vi "Test DQMH Power Requests API.vi"() -> ()   [LabVIEW 2024]
doc: "DQMH Power Requests API Tester.\n\n<b>Note:</b> This VI was modified by the <b>Validate DQMH Module</b> tool to upgrade it to the DQMH 5.0 approach to only call the Stop Module.vi at the end of the tester if the module wasn't originally running when the tester started.\n\n<b>Note:</b> This VI was modified by the <b>Validate DQMH Module</b> tool to add the 'Show Main VI Diagram on Init' functionality included in DQMH 6.1.\n\n<b>Note:</b> This VI was modified by the <b>Validate DQMH Module</b> tool to upgrade its Error Reported event frame to use an improved mechanism for displaying error information.\n\n<b>Note:</b> This VI was modified by the <b>Validate DQMH Module</b> tool to remove code to stop the main loop on error, and instead display the most recent error on the tester front panel."
uses:
  <vilib>/Utility/error.llb/DialogType.ctl
  DQMH Power Requests.lvlib
panel:
  out "last error":errorcluster
  in  "Show Main VI Diagram on Init (F)":bool
  in  "Display Required":bool
  in  "System Required":bool
  in  "Create Request":bool
  in  "Show Block Diagram":bool
  in  "Stop Module":bool
  in  "Start Module":bool
  in  "Hide Module Panel":bool
  in  "Show Module Panel":bool
  out "Status":string
  out "Module Running?":bool
  # "This VI tests the API for the Module."
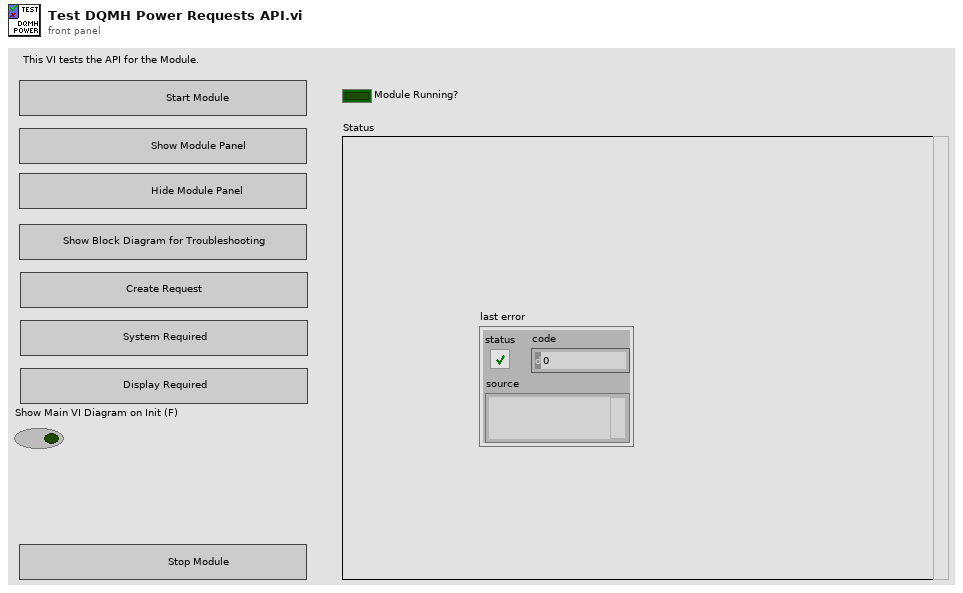
[diagram p1: front panel]
types:
  T1 = typedef "DQMH Power Requests.lvlib/Broadcast Events--cluster.ctl" = cluster{"Module Did Init":refnum<user-event>, "Status Updated":refnum<user-event>, "Error Reported":refnum<user-event>, "Module Did Stop":refnum<user-event>, "Update Module Execution Status":refnum<user-event>}
  T2 = typedef "DialogType.ctl" = u16
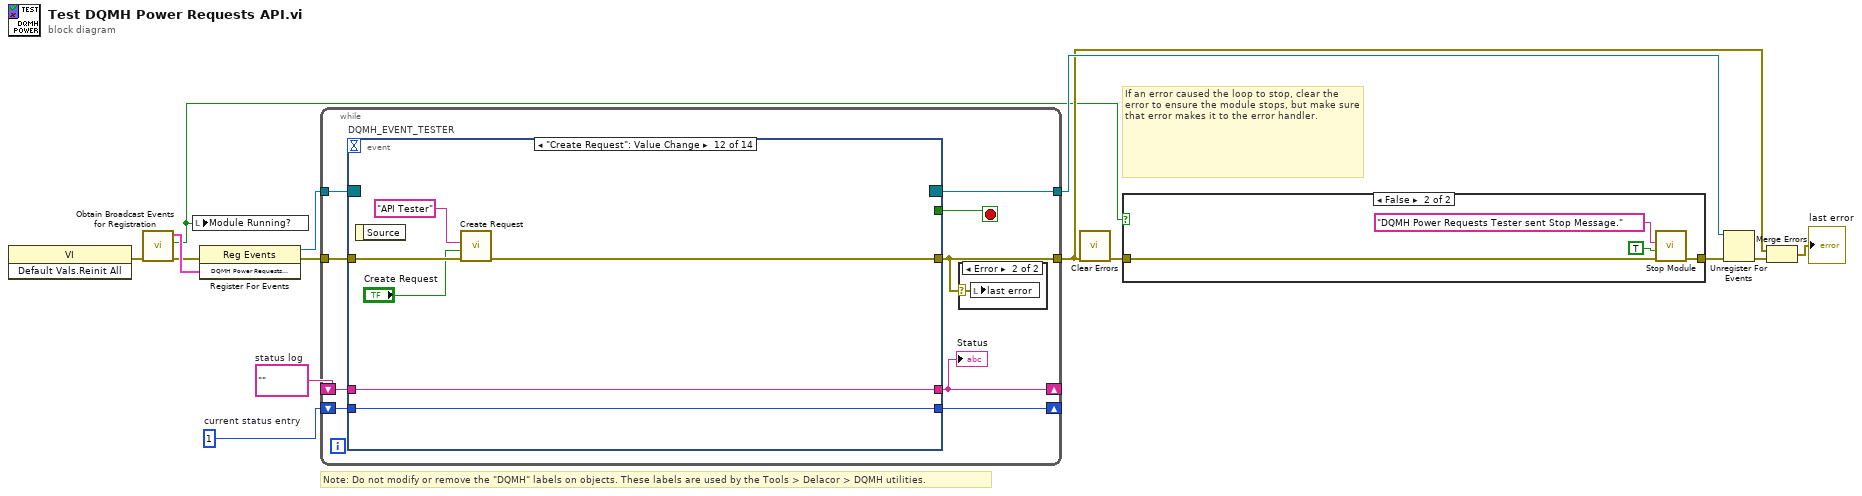
[diagram p0: block diagram]
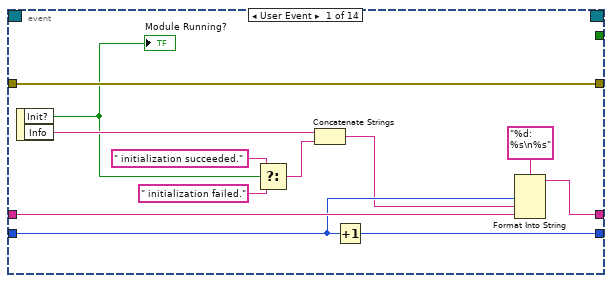
[diagram p4: hidden frame]
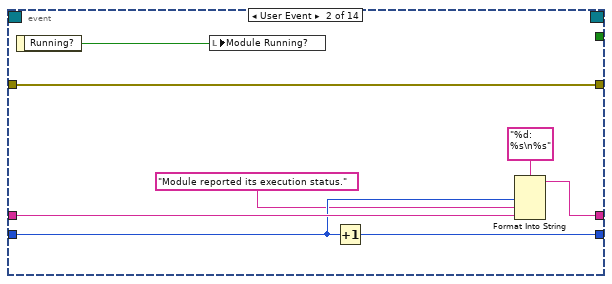
[diagram p5: hidden frame]
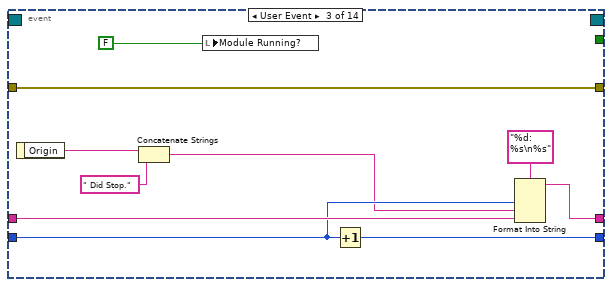
[diagram p6: hidden frame]
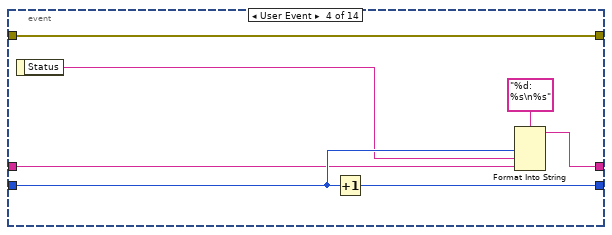
[diagram p7: hidden frame]
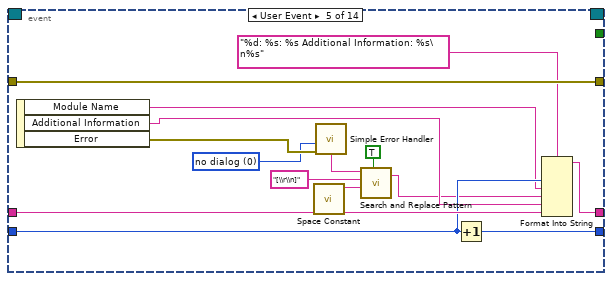
[diagram p8: hidden frame]
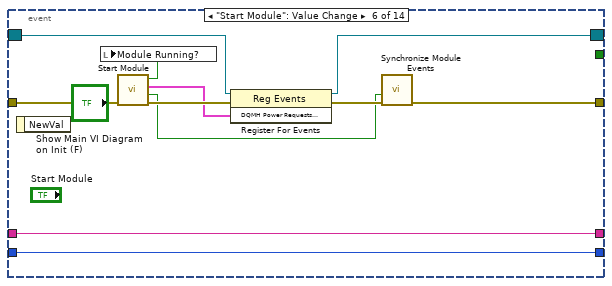
[diagram p9: hidden frame]
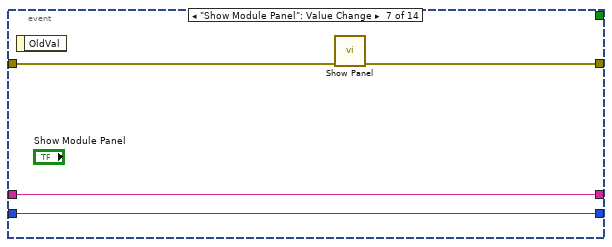
[diagram p10: hidden frame]
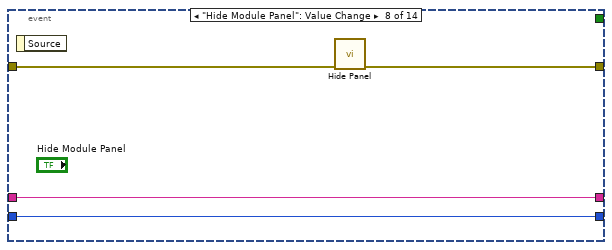
[diagram p11: hidden frame]
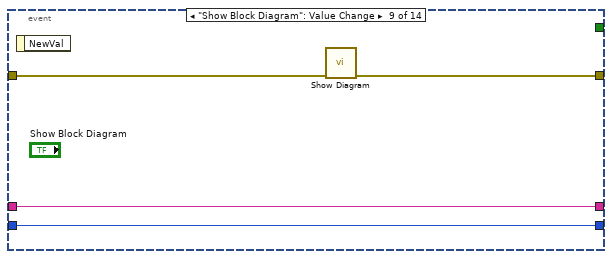
[diagram p12: hidden frame]
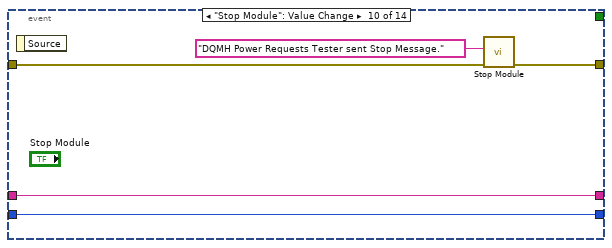
[diagram p13: hidden frame]
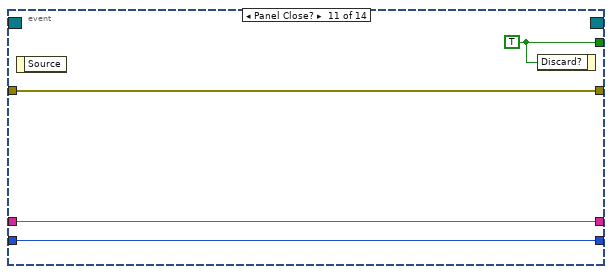
[diagram p14: hidden frame]
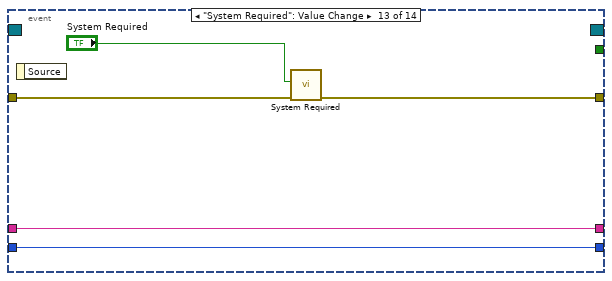
[diagram p15: hidden frame]
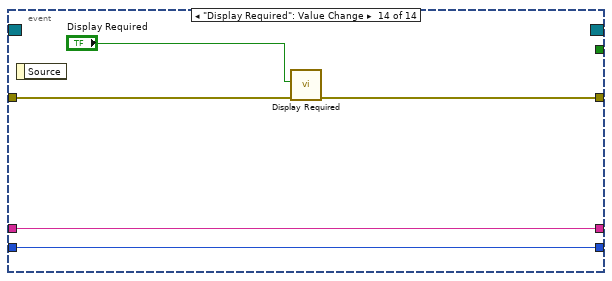
[diagram p16: hidden frame]
diagram:
  w11 = 1  # current status entry
  w12 = ""  # status log
  # "If an error caused the loop to stop, clear the error to ensure the module stops, but make sure that error makes it to the error handler."
  # "Note: Do not modify or remove the \"DQMH\" labels on objects. These labels are used by the Tools > Delacor > DQMH utilities."
  n1 = invoke class="VI" method="Default Vals.Reinit All"() -> (error out=w3:errorcluster)  [unwired: 3 in, 2 out]
  n2 = call "Obtain Broadcast Events for Registration.vi"("error in (no error)"=w3) -> ("error out"=w2:errorcluster, "Already running?"=w4:bool, "DQMH Power Requests Broadcast Events"=w9:T1)  [unwired: 8 in]
  n3 = local write "Module Running?"(w4) -> ()
  n4 = register-events(error in=w2, w9) -> (reference out=w8:refnum<event-registration>, error out=w10:errorcluster)  [unwired: 1 in]
  n5 = while {
    tunnel: w8 -> [w23]
    tunnel: [w16] -> w5
    shift-right: [w19] -> _
    shift-left: w12 -> [w21]
    shift-right: [w20] -> _
    shift-left: w11 -> [w22]
    tunnel: w10 -> [w18]
    tunnel: [w17] -> w7
    stop <- w15 stop-if-true
    n6 = event "DQMH_EVENT_TESTER" shown="[11] \"Create Request\": Value Change" {
      selector: w23 -> [_ _ _ _ _ w82 _ _ _ _ _ _ _ _]
      dyn-events: [_ _ _ _ _ w81 _ _ _ _ _ _ _ _] -> w17
      timeout: _ -> [_ _ _ _ _ _ _ _ _ _ _ _ _ _]
      tunnel: [_ _ _ _ _ _ _ _ _ _ w109 _ _ _] -> w15
      tunnel: [w36 w38 w45 w55 w76 w80 w92 w96 w97 w103 w106 w110 w117 w122] -> w16
      tunnel: w22 -> [w33 w42 w52 w58 w73 w85 w90 w94 w98 w104 w107 w113 w118 w123]
      tunnel: w21 -> [w34 w43 w53 w57 w75 w86 w91 w95 w99 w105 w108 w114 w119 w124]
      tunnel: [w31 w40 w50 w59 w74 w86 w91 w95 w99 w105 w108 w114 w119 w124] -> w19
      tunnel: [w32 w41 w51 w61 w72 w85 w90 w94 w98 w104 w107 w113 w118 w123] -> w20
      tunnel: w18 -> [w36 w38 w45 w55 w76 w79 w89 w93 w100 w101 w106 w115 w120 w125]
      event User Event {
        n7 = event-data() -> ("Init?"=w28:bool, "Info"=w30:string)  [unwired: 1 in]
        "Module Running?" <- w28
        n8 = Select(t=" initialization succeeded.", s=w28, f=" initialization failed.") -> (s? t:f=w25:string)
        n9 = Concatenate Strings(w30, w25) -> (w29:string)
        n10 = Increment(x=w33) -> (x+1=w32:i32)
        n11 = Format Into String(format string="%d: %s\n%s", w33, w29, w34) -> (resulting string=w31:string)  [unwired: 2 in, 1 out]
      }
      event User Event {
        n12 = event-data() -> ("Running?"=w37:bool)  [unwired: 1 in]
        n13 = local write "Module Running?"(w37) -> ()
        n14 = Increment(x=w42) -> (x+1=w41:i32)
        n15 = Format Into String(format string="%d: %s\n%s", w42, "Module reported its execution status.", w43) -> (resulting string=w40:string)  [unwired: 2 in, 1 out]
      }
      event User Event {
        n16 = event-data() -> ("Origin"=w49:string)  [unwired: 1 in]
        n17 = Concatenate Strings(w49, " Did Stop.") -> (w48:string)
        n18 = local write "Module Running?"(FALSE ("Module Did Init?")) -> ()
        n19 = Increment(x=w52) -> (x+1=w51:i32)
        n20 = Format Into String(format string="%d: %s\n%s", w52, w48, w53) -> (resulting string=w50:string)  [unwired: 2 in, 1 out]
      }
      event User Event {
        n21 = event-data() -> ("Status"=w56:string)  [unwired: 1 in]
        n22 = Increment(x=w58) -> (x+1=w61:i32)
        n23 = Format Into String(format string="%d: %s\n%s", w58, w56, w57) -> (resulting string=w59:string)  [unwired: 2 in, 1 out]
      }
      event User Event {
        w68 = T2 0 items=["no dialog", "OK message", "continue or stop message", "OK message + warnings", "continue/stop + warnings"] ("type of dialog (OK msg:1)")
        n24 = event-data() -> ("Module Name"=w69:string, "Additional Information"=w70:string, "Error"=w71:errorcluster)  [unwired: 1 in]
        n25 = call <vilib>:"Space Constant.vi"() -> ("String"=w64:string)
        n26 = call <vilib>:"Simple Error Handler.vi"("type of dialog (OK msg:1)"=w68, "error in (no error)"=w71) -> ("message"=w67:string)  [unwired: 3 in, 4 out]
        n27 = call <vilib>:"Search and Replace Pattern.vi"("string"=w67, "regular expression (\"\")"="[\\r\\n]" ("regular expression (\"\")"), "replace string (\"\")"=w64, "replace all? (F)"=TRUE ("replace all CR/LF with spaces")) -> ("result string"=w66:string)  [unwired: 1 in, 1 out]
        n28 = Increment(x=w73) -> (x+1=w72:i32)
        n29 = Format Into String(format string="%d: %s: %s Additional Information: %s\n%s", w73, w69, w66, w70, w75) -> (resulting string=w74:string)  [unwired: 2 in, 1 out]
      }
      event "Start Module": Value Change {
        n30 = event-data() -> ()  [unwired: 1 in, 1 out]
        n31 = call "Start Module.vi"("Show Main VI Diagram on Init (F)"="Show Main VI Diagram on Init (F)", "error in (no error)"=w79) -> ("error out"=w87:errorcluster, "Wait for Event Sync?"=w84:bool, "DQMH Power Requests Broadcast Events"=w83:T1, "Module Was Already Running?"=w78:bool)  [unwired: 6 in]
        n32 = local write "Module Running?"(w78) -> ()
        n33 = register-events(reference=w82, error in=w87, w83) -> (reference out=w81:refnum<event-registration>, error out=w88:errorcluster)
        n34 = call "Synchronize Module Events.vi"("error in (no error)"=w88, "Wait for Event Sync?"=w84) -> ("error out"=w80:errorcluster)  [unwired: 9 in]
      }
      event "Show Module Panel": Value Change {
        n35 = event-data() -> ()  [unwired: 1 in, 1 out]
        n36 = call "Show Panel.vi"("error in (no error)"=w89) -> ("error out"=w92:errorcluster)  [unwired: 10 in]
      }
      event "Hide Module Panel": Value Change {
        n37 = event-data() -> ()  [unwired: 1 in, 1 out]
        n38 = call "Hide Panel.vi"("error in (no error)"=w93) -> ("error out"=w96:errorcluster)  [unwired: 10 in]
      }
      event "Show Block Diagram": Value Change {
        n39 = event-data() -> ()  [unwired: 1 in, 1 out]
        n40 = call "Show Diagram.vi"("error in (no error)"=w100) -> ("error out"=w97:errorcluster)  [unwired: 10 in]
      }
      event "Stop Module": Value Change {
        n41 = event-data() -> ()  [unwired: 1 in, 1 out]
        n42 = call "Stop Module.vi"("error in (no error)"=w101, "Origin"="DQMH Power Requests Tester sent Stop Message.") -> ("error out"=w103:errorcluster)  [unwired: 9 in]
      }
      event Panel Close? {
        w109 = TRUE ("Discard?")
        n43 = event-data() -> ()  [unwired: 1 in, 1 out]
        n44 = event-data("Discard?"=w109) -> ()  [unwired: 1 in, 1 out]
      }
      event "Create Request": Value Change {
        n45 = event-data() -> ()  [unwired: 1 in, 1 out]
        n46 = call "Create Request.vi"("error in (no error)"=w115, "Create"="Create Request", "Simple Reason String"="API Tester") -> ("error out"=w110:errorcluster)  [unwired: 6 in, 2 out]
      }
      event "System Required": Value Change {
        n47 = event-data() -> ()  [unwired: 1 in, 1 out]
        n48 = call "System Required.vi"("error in (no error)"=w120, "Create"="System Required") -> ("error out"=w117:errorcluster)  [unwired: 7 in, 2 out]
      }
      event "Display Required": Value Change {
        n49 = event-data() -> ()  [unwired: 1 in, 1 out]
        n50 = call "Display Required.vi"("error in (no error)"=w125, "Create"="Display Required") -> ("error out"=w122:errorcluster)  [unwired: 7 in, 2 out]
      }
    }
    "Status" <- w19
    n51 = case "DQMH_TESTER_ERROR_LOCAL" shown="Error" w16 {
      selector: w16 -> [_ w24]
      frame No Error {
      }
      frame Error {
        n52 = local write "last error"(w24) -> ()
      }
    }
  }
  n53 = call <vilib>:"Clear Errors.vi"("error in (no error)"=w5) -> ("error out"=w6:errorcluster)  [unwired: 5 in, 1 out]
  n54 = case shown="False" w4 {
    tunnel: [w126 w130] -> w13
    tunnel: w6 -> [w126 w127]
    frame True {
    }
    frame False {
      n55 = call "Stop Module.vi"("error in (no error)"=w127, "Wait for Module to Stop? (F)"=TRUE ("Wait for Module to stop?"), "Origin"="DQMH Power Requests Tester sent Stop Message.") -> ("error out"=w130:errorcluster)  [unwired: 8 in]
    }
  }
  n56 = Unregister For Events(event registration refnum=w7, error in=w13) -> (error out=w14:errorcluster)
  n57 = Merge Errors(w5, w14) -> (→"last error":errorcluster)
